vi "Get_ADAM_Ch_names_client.vi"(1 "Channel names set":T1) -> (0 "Ch names":string[](array[string]))   [LabVIEW 2010]
doc: "This is an example of using features of the VI Server as a client. It shows how you might browse from one or more applications that may be exporting data from one or more data stations. \n\nThe example shows how to query a server for its list of exported VIs, how to get references to the VIs, and how call them with the Call By Reference function."
uses:
  Sub VIs/ADAM Controls/Channel_names.ctl
  Anemometry/Anemometry Sub Vis/Controls/Global_mode.ctl
  Sub VIs/ADAM Controls/Channel_State.ctl
  Anemometry/Anemometry Sub Vis/Globals/Preference_global.vi
panel:
  in  "Server type":refnum<vi>
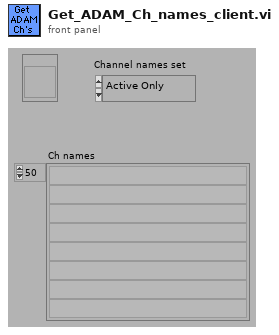
[diagram p1: front panel]
types:
  T1 = typedef "Channel_names.ctl" = enum16{"Active Only", "Active + Off", "All Channels"}
  T2 = typedef "Server_Comms.ctl" = enum16{"Server Link Healthy", "Do Not Link To Server"}
  T3 = typedef "Global_mode.ctl" = enum16{"Read Global", "Load Global From File", "Write Global to File"}
  T4 = typedef "Channel_State.ctl" = enum16{"On", "Off", "Always On", "Always Off"}
  T5 = typedef "Ch_description_ADAM.ctl" = cluster{"Ch Name":string, "Type":T6, "Function":T7, "Ch State":T4, "Calibration type":T8, "A":dbl, "B":dbl, "C":dbl, "D":dbl, "Comments":string, "Address":T9, "String":string, "Duty":u16}
  T6 = typedef "Module_type_ADAM.ctl" = enum16{"4011", "4012", "4013", "4014", "4016", "4017", "4018", "4021", "4050", "4052", "4053", "4060", "4080", "5000", "5017", "5018", "5024", "5051", "5056", "5060", "6060", "Tracker", "WEST", "GILL", "JEM", "VICI", "Vaisala", "DRUCK", "Run VI Named:", "IR2100", "PPT", "Comparator", "VIRTUAL", "Hold Value", "Read A", "Read Ch", "Coded", "Client Info", "Web Client", "X10", "Test"}
  T7 = typedef "Function_ADAM.ctl" = enum16{"Analogue Input", "Digital Input", "Event counter", "Event rate", "Analogue Output", "Digital Output", "Relay Output"}
  T8 = typedef "Calib_type_ADAM.ctl" = enum16{"Raw", "Bx + A", "Cx^2 + Bx + A", "Dx^3 + Cx^2 + Bx + A", "In Band", "Hi-Tec Q", "Hi-Tec M_dot", "Text"}
  T9 = typedef "Address.ctl" = cluster{"Main":i32, "Ch.":i32, "Sub":i32, "Port Name":string}
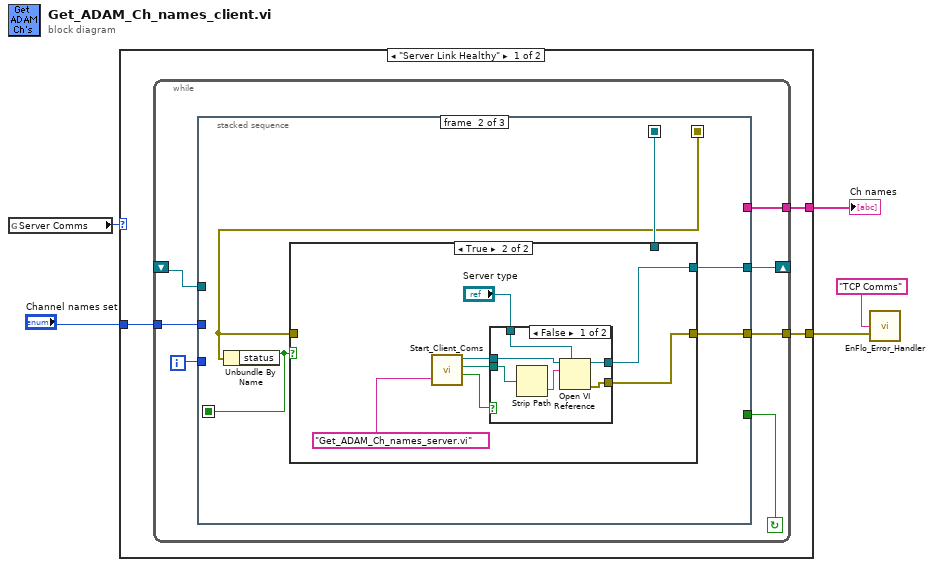
[diagram p0: block diagram]
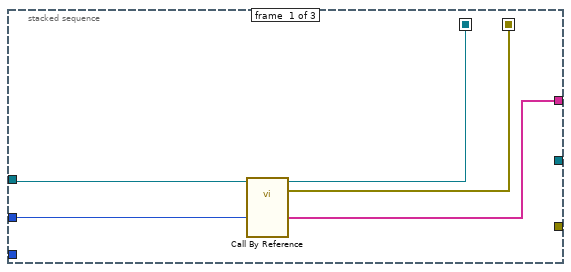
[diagram p2: hidden frame]
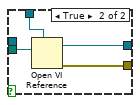
[diagram p4: hidden frame]
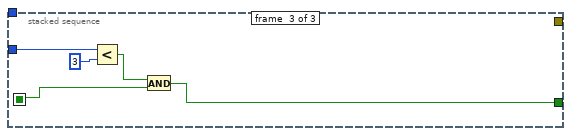
[diagram p5: hidden frame]
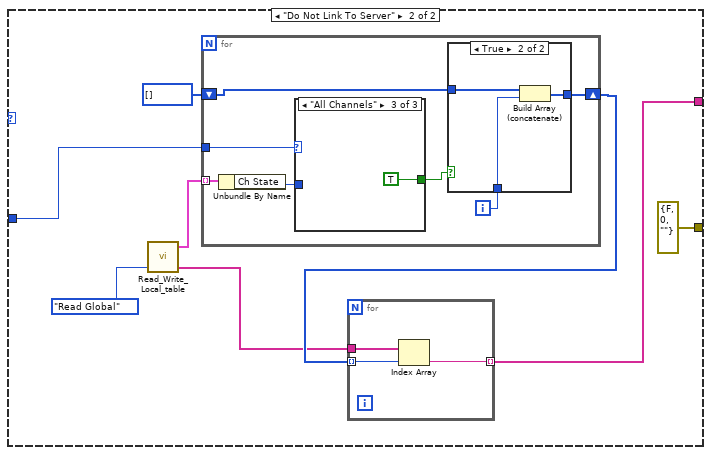
[diagram p6: hidden frame]
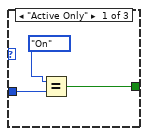
[diagram p8: hidden frame]
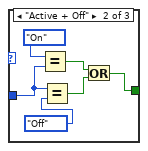
[diagram p9: hidden frame]
diagram:
  n1 = global read "Preference_global.vi" "Server Comms"() -> (w4:T2)
  n2 = case shown="\"Server Link Healthy\"" w4 {
    tunnel: [w8 w50] -> w5
    tunnel: [w7 errorcluster {"status"=FALSE, "code"=0, "source"=""} ("Error IO")] -> w3
    tunnel: "Channel names set" -> [w6 w54]
    frame "Server Link Healthy" {
      n3 = while {
        tunnel: [w10] -> w7
        tunnel: [w11] -> w8
        shift-left: _ -> [w15]
        shift-right: [w14] -> _
        tunnel: w6 -> [w9]
        i -> [w13]
        stop <- w12 continue-if-true
        n4 = stacked-sequence {
          seq-local: [w18 _ _] -> [_ w24 _]
          seq-local: [w17 _ _] -> [_ w21 _]
          seq-local: [_ w23 _] -> [_ _ w46]
          tunnel: w15 -> [w20 _ _]
          tunnel: [_ w25 _] -> w14
          tunnel: w13 -> [_ _ w47]
          tunnel: [_ _ w45] -> w12
          tunnel: [w19 _ _] -> w11
          tunnel: [_ w22 _] -> w10
          tunnel: w9 -> [w16 _ _]
          frame #0 {
            n5 = call-by-ref "?"(reference=w20, "Channel names set"=w16) -> (reference out=w18:refnum<vi>, error out=w17:errorcluster, "Ch names"=w19:string[])  [unwired: 1 in]
          }
          frame #1 {
            n6 = Unbundle By Name(w21) -> ("status"=w23:bool)
            n7 = case shown="True" w23 {
              tunnel: [w27 w30] -> w25
              tunnel: w24 -> [w27 _]
              tunnel: [w26 w28] -> w22
              tunnel: w21 -> [w26 _]
              frame False {
              }
              frame True {
                n8 = call "Start_Client_Coms.vi"("VI name to run on server"="Get_ADAM_Ch_names_server.vi") -> ("LabVIEW application reference"=w32:refnum<vi>, "Checked VI name"=w33:path, "Local Call"=w31:bool)  [unwired: 1 in, 1 out]
                n9 = case shown="False" w31 {
                  tunnel: [w37 w44] -> w30
                  tunnel: "Server type" -> [w36 w43]
                  tunnel: w33 -> [w40 w42]
                  tunnel: w32 -> [w35 _]
                  tunnel: [w38 w41] -> w28
                  frame False {
                    n10 = Strip Path(path=w40) -> (name=w39:string)  [unwired: 1 out]
                    n11 = Open VI Reference(type specifier VI Refnum (for type only)=w36, application reference (local)=w35, vi path=w39) -> (vi reference=w37:refnum<vi>, error out=w38:errorcluster)  [unwired: 1 in, 2 out]
                  }
                  frame True {
                    n12 = Open VI Reference(type specifier VI Refnum (for type only)=w43, vi path=w42) -> (vi reference=w44:refnum<vi>, error out=w41:errorcluster)  [unwired: 1 in, 3 out]
                  }
                }
              }
            }
          }
          frame #2 {
            n13 = Less?(x=w47, y=3) -> (x < y?=w49:bool)
            n14 = And(x=w49, y=w46) -> (x .and. y?=w45:bool)
          }
        }
      }
    }
    frame "Do Not Link To Server" {
      n15 = call "Read_Write_Local_table.vi"("Mode"=Global_mode."Read Global") -> ("Ch Names"=w51:string[], "Channels Descriptions Out"=w55:T5[])  [unwired: 2 in, 1 out]
      n16 = for {
        tunnel: w55 -> [w67] mode=indexing
        tunnel: w54 -> [w66]
        shift-right: [w62] -> w52
        shift-left: i32[] [] -> [w61]
        i -> [w63]
        n17 = Unbundle By Name(w67) -> ("Ch State"=w65:T4)
        n18 = case shown="\"All Channels\"" w66 {
          tunnel: w65 -> [w74 w79 _]
          tunnel: [w72 w75 TRUE] -> w64
          frame "Active Only" {
            n19 = Equal?(x=Channel_State."On" ("Ch State"), y=w74) -> (x = y?=w72:bool)
          }
          frame "Active + Off" {
            n20 = Equal?(x=Channel_State."On" ("Ch State"), y=w79) -> (x = y?=w76:bool)
            n21 = Equal?(x=w79, y=Channel_State."Off" ("Ch State")) -> (x = y?=w77:bool)
            n22 = Or(x=w76, y=w77) -> (x .or. y?=w75:bool)
          }
          frame "All Channels" {
          }
        }
        n23 = case shown="True" w64 {
          tunnel: w63 -> [_ w71]
          tunnel: [w68 w70] -> w62
          tunnel: w61 -> [w68 w69]
          frame False {
          }
          frame True {
            n24 = Build Array (concatenate)(w69, w71) -> (w70:i32[])
          }
        }
      }
      n25 = for {
        tunnel: w52 -> [w60] mode=indexing
        tunnel: w51 -> [w59]
        tunnel: [w58] -> w50 mode=indexing
        n26 = Index Array(array=w59, index=w60) -> (element=w58:string)
      }
    }
  }
  "Ch names" <- w5
  n27 = call "EnFlo_Error_Handler.vi"("error in (no error)"=w3, "Error Type"="TCP Comms") -> ()  [unwired: 1 in, 3 out]
